vi "update_past_RowData.vi"(10 "RowData input":T1, 11 "Clarified turbidity (mg/L)":dbl) -> (3 "RowData output":T1)   [LabVIEW 2019]
uses:
  RowData_Type.ctl
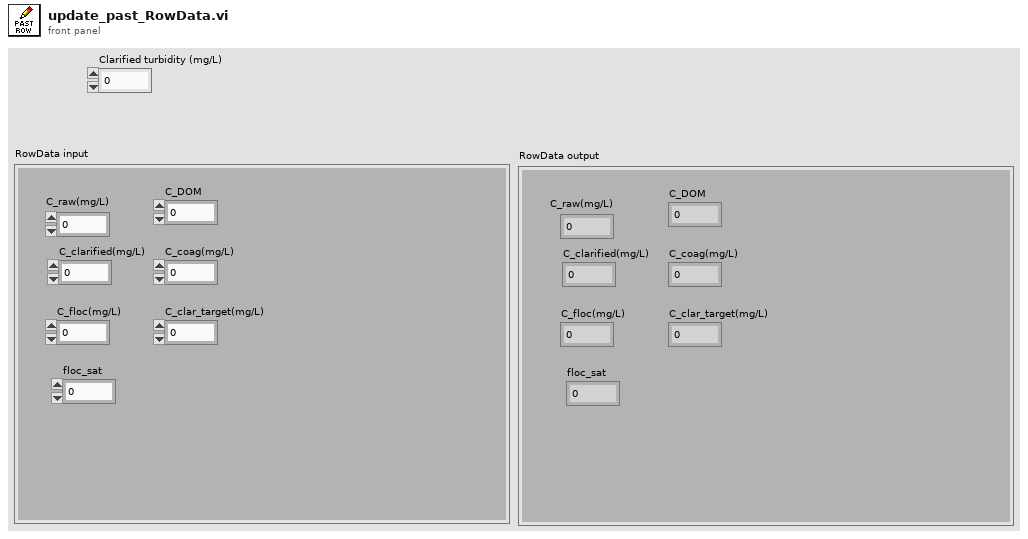
[diagram p1: front panel]
types:
  T1 = typedef "RowData_Type.ctl" = cluster{"C_raw(mg/L)":dbl, "C_clarified(mg/L)":dbl, "C_floc(mg/L)":dbl, "floc_sat":dbl, "C_DOM":dbl, "C_coag(mg/L)":dbl, "C_clar_target(mg/L)":dbl}
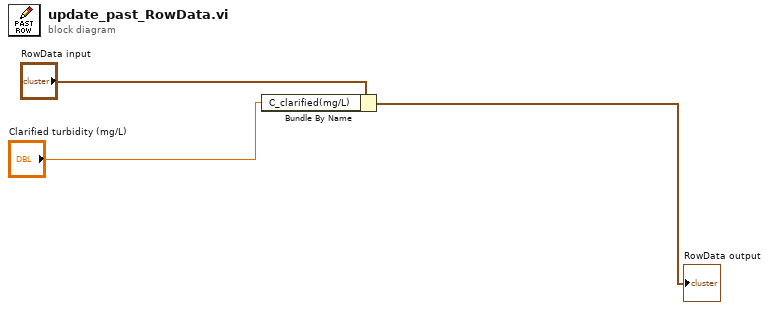
[diagram p0: block diagram]
diagram:
  n1 = Bundle By Name(cluster="RowData input", "C_clarified(mg/L)"="Clarified turbidity (mg/L)") -> (→"RowData output":T1)
